vi "CurrentPosition.vi"() -> ()   [LabVIEW 2012]
panel:
  in  "Current position":dbl[](array[numeric])
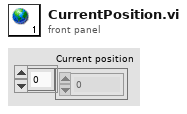
[diagram p1: front panel]
diagram:
